vi "remove nan from array (subVI).vi"(1 "array":dbl[](array[numeric])) -> (0 "nan-free array":dbl[](array[numeric]))   [LabVIEW 2021]
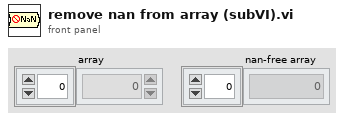
[diagram p1: front panel]
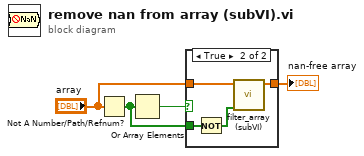
[diagram p0: block diagram]
diagram:
  n1 = Not A Number/Path/Refnum?(number/path/refnum="array") -> (NaN/Path/Refnum?=w3:bool[])
  n2 = Or Array Elements(Boolean array=w3) -> (logical OR=w4:bool)
  n3 = case shown="True" w4 {
    tunnel: w3 -> [_ w9]
    tunnel: "array" -> [w5 w8]
    tunnel: [w5 w6] -> w1
    frame False {
    }
    frame True {
      n4 = Not(x=w9) -> (.not. x?=w7:bool[])
      n5 = call "filter_array (subVI).vi"("filter"=w7, "array"=w8) -> ("filtered array"=w6:dbl[])  [unwired: 9 in]
    }
  }
  "nan-free array" <- w1
